vi "File saving using labview.vi"() -> ()   [LabVIEW 2018]
panel:
  in  "file path (use dialog) 2":path
  out "TEXT 2":string
  in  "file path (use dialog)":path
  in  "TEXT":string
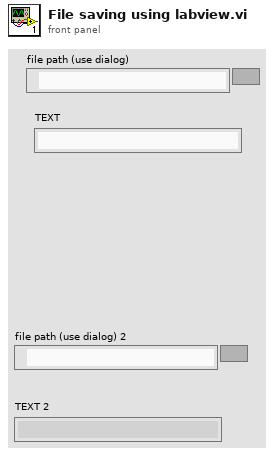
[diagram p1: front panel]
types:
  T1 = enum16{"open", "replace", "create", "open or create", "replace or create", "replace or create with confirmation"}
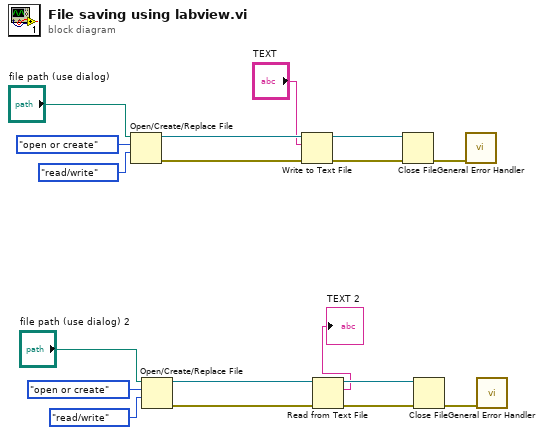
[diagram p0: block diagram]
diagram:
  n1 = Open/Create/Replace File(file path (use dialog)="file path (use dialog)", operation (0:open)=T1."open or create", access (0:read/write)=enum16{"read/write", "read-only", "write-only"}."read/write") -> (refnum out=w15:refnum<file>, error out=w13:errorcluster)  [unwired: 3 in, 1 out]
  n2 = Open/Create/Replace File(file path (use dialog)="file path (use dialog) 2", operation (0:open)=T1."open or create", access (0:read/write)=enum16{"read/write", "read-only", "write-only"}."read/write") -> (refnum out=w6:refnum<file>, error out=w4:errorcluster)  [unwired: 3 in, 1 out]
  n3 = Write to Text File(file (use dialog)=w15, text="TEXT", error in=w13) -> (refnum out=w14:refnum<file>, error out=w12:errorcluster)  [unwired: 1 in, 1 out]
  n4 = Read from Text File(file (use dialog)=w6, error in=w4) -> (refnum out=w5:refnum<file>, text=→"TEXT 2":string, error out=w3:errorcluster)  [unwired: 2 in, 1 out]
  n5 = Close File(refnum=w14, error in=w12) -> (error out=w11:errorcluster)  [unwired: 1 out]
  n6 = Close File(refnum=w5, error in=w3) -> (error out=w2:errorcluster)  [unwired: 1 out]
  n7 = call <vilib>:"General Error Handler.vi"("error in (no error)"=w11) -> ()  [unwired: 10 in, 5 out]
  n8 = call <vilib>:"General Error Handler.vi"("error in (no error)"=w2) -> ()  [unwired: 10 in, 5 out]
